vi "Get Export Setup.vi"(8 "error in (no error)":errorcluster, 11 "Map":T1) -> (0 "error out":errorcluster, 1 "Export Setup":T2[](array[typedef]), 3 "Map Out":T1)   [LabVIEW 2015, in "ConfigHelper.lvlib"]
uses:
  Control_Export Setup.ctl
  <vilib>/addons/PointValueMap/controls/PointMap.ctl
  <vilib>/addons/PointValueMap/subVIs/Point_Read_variant.vi
  ConfigHelper.lvlib
  <vilib>/addons/PointValueMap/PointValueMap.lvlib
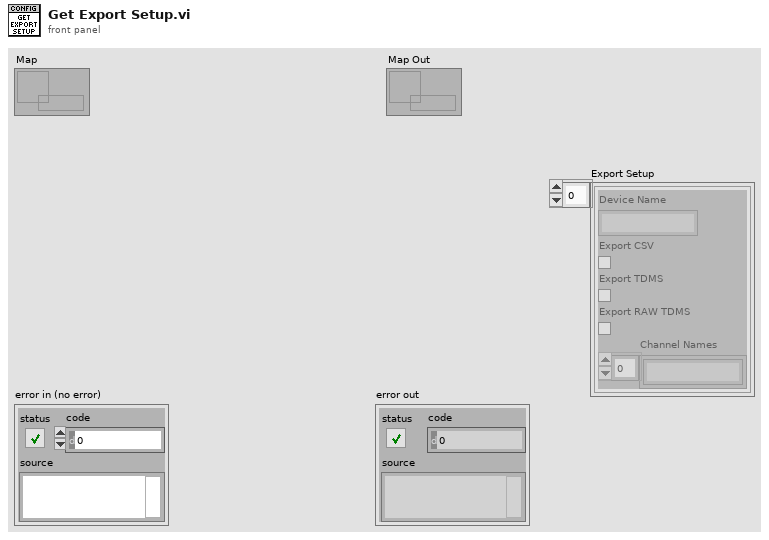
[diagram p1: front panel]
types:
  T1 = typedef "PointValueMap.lvlib/PointMap.ctl" = refnum<data-value>
  T2 = typedef "ConfigHelper.lvlib/Control_Export Setup.ctl" = cluster{"Device Name":string, "Export CSV":bool, "Export TDMS":bool, "Export RAW TDMS":bool, "Channel Names":string[]}
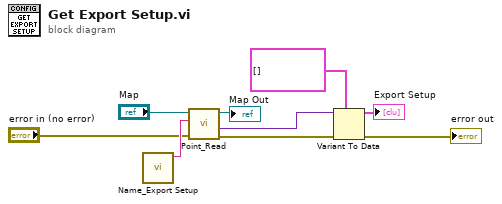
[diagram p0: block diagram]
diagram:
  n1 = call "Name_Export Setup.vi"() -> ("Name"=w5:string)  [unwired: 11 in]
  n2 = call-poly <vilib>:"Point_Read.vi"("Error In"="error in (no error)", "Tag"=w5, "Map"="Map") -> ("Error Out"=w9:errorcluster, "Value"=w8:variant, "Map Out"=→"Map Out":T1)  [unwired: 3 in, 3 out]
  n3 = Variant To Data(error in=w9, type=T2[] [], Variant=w8) -> (data=→"Export Setup":T2[], error out=→"error out":errorcluster)
